vi "AlliGator Phasor Plot Context Menu Handler.vi"(8 "Error In":errorcluster, 11 "Image Event":T1) -> (0 "Error Out":errorcluster, 1 "Message":string, 3 "AlliGator Actions":T4[](array[typedef]))   [LabVIEW 2021, in "AlliGator Phasor Plot.lvlib"]
doc: "Phasor Plot image context menu handler."
uses:
  AlliGator Phasor Plot.lvlib
  Action Engine/AlliGator Q Element.ctl
  Action Engine/AlliGator Q Event.ctl
  Image/Image Display Event.ctl
  Image/Image Control Refnum.ctl
  <vilib>/Utility/miscctls.llb/LVPoint32TypeDef.ctl
  Image/Image Display to Clipboard Options.ctl
  Settings/AlliGator Phasor Plot Graphics Options.ctl
  Settings/AlliGator Settings List.ctl
  ROIs/AlliGator ROI Manager Actions.ctl
  ROIs/AlliGator Selected ROI.ctl
  Image/Image Control ROI Description.ctl
  GUI/AlliGator Windows List.ctl
  AlliGator Phasor Harmonic Manager Actions.ctl
  Phasor Plot Color Map/AlliGator Phasor Color Map Picker.vi
  Variant/Variant to Data/Variant to Boolean.vi
  ROIs/AlliGator Phasor Plot ROI Manager.vi
  Action Engine/AlliGator Action Engine.lvlib
  Image/Image.lvlib
  Settings/AlliGator Settings.lvlib
  Variant/Variant to Data/Variant to Data.lvlib
  Utilities/Utilities.lvlib
  Phasor Plot Color Map/AlliGator Phasor Plot Color Map.lvlib
  ROIs/AlliGator ROIs.lvlib
  GUI/AlliGator GUI.lvlib
  AlliGator Phasor Harmonics.lvlib
  Notebook/Notebook.lvlib
panel:
  # "see the AlliGator License on the block diagram (Ctrl+E or Window:Show Block Diagram)"
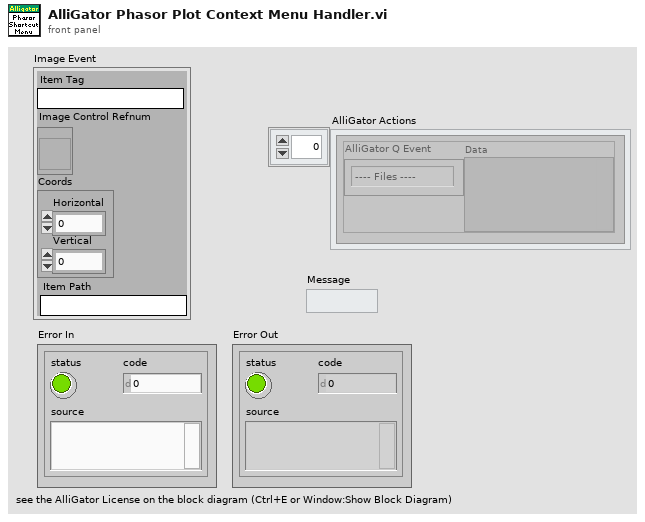
[diagram p1: front panel]
types:
  T1 = typedef "Image.lvlib/Image Display Event.ctl" = cluster{"Item Tag":string, "Image Control Refnum":T2, "Coords":T3, "Item Path":string}
  T2 = typedef "Image.lvlib/Image Control Refnum.ctl" = refnum<vi>
  T3 = typedef "LVPoint32TypeDef.ctl" = cluster{"Horizontal":i32, "Vertical":i32}
  T4 = typedef "AlliGator Action Engine.lvlib/AlliGator Q Element.ctl" = cluster{"AlliGator Q Event":T5, "Data":variant}
  T5 = typedef "AlliGator Action Engine.lvlib/AlliGator Q Event.ctl" = enum16{"---- Files ----", "Files:Set Batch Export Files To Save", "Files:Set Dataset Loading & Pre-processing Options", "Files:Check #Frames in Dataset", "Files:Increment Frame Index", "Files:Open Mask Image", "Files:Open White Light Image", "Files:Open Single Dataset", "Files:New Folder of Folders Selected", "Files:Load File (all Types)_Scriptable", "Files:Move Flattened Series to Folders Series", "Files:Select Folder", "Files:Load FLI Dataset", "Files:Load Swiss SPAD 1 Dataset", "Files:Load Swiss SPAD 2 Dataset", "Files:Load .sdt FLI Dataset", "Files:Load .ptu FLI Dataset", "Files:Load .bin FLI Dataset", "Files:Load Single Gate Image Folder", "Files:Load I/m/phi Dataset (deprecated)", "Files:Load Single Image", "Files:Subtract Background File", "Files:Export FLI Dataset", "Files:Load HDF5 FLI Dataset", "Files:Set Destination File Path", "Files:Save Mask Image", "Files:Batch Conversion", "Files:New Folder Selected", "Files:Close FLI Dataset", "Files:Close FLI Dataset Series", "Files:Close White Light Image", "Files:Close Mask Image", "---- FLI Dataset ----", "FLI Dataset:Channel Arithmetic", "FLI Dataset:Export Average Lifetime Map as ASCII", "FLI Dataset:Export User-Defined Quantity Map as ASCII", "FLI Dataset:Python Function FLI Dataset Event", "FLI Dataset:ROI Analysis", "FLI Dataset:Tilted Logistic Square Gated IRF Characteristics Map", "FLI Dataset:Logistic Square Gated IRF Characteristics Map", "FLI Dataset:Square Gated IRF Characteristics Map", "FLI Dataset:Multi-ROI Single-Pixel Phasor Analysis", "FLI Dataset:Multi-ROI Single-Pixel NLSF Analysis", "FLI Dataset:All ROIs IRF Extraction", "FLI Dataset:All ROIs Decay Fit Non-Interactive (Fast + Individual IRF)", "FLI Dataset:All ROIs Phasor Analysis", "FLI Dataset:All ROIs Decay Fit", "FLI Dataset:Fluorescence Decay Statistics", "FLI Dataset:Update Decay Statistics Graph", "FLI Dataset:Get Decay from ROI", "FLI Dataset:All ROIs Average Lifetimes", "---- FLI Dataset Series ----", "FLI Dataset Series:Sum All Datasets in Series", "FLI Dataset Series:Add Dataset to Accumulated Dataset", "FLI Dataset Series:Display Accumulated Dataset", "FLI Dataset Series:Clear Dataset Series Sum", "FLI Dataset Series:Time-Series Analysis (NLSF)", "FLI Dataset Series:Time-Series Analysis (Phasor)", "---- Image ----", "Image:Update Image Profile Plots", "Image:Image Histogram Cursor Move", "Image:Image Histogram", "Image:Image Contrast", "Image:Set Image Histogram Cursor Move Flag", "Image:Clear Image Overlay", "Image:Use ROI as Search Area", "Image:Set ROI Diameter", "Image:Save Image Data as TIFF", "Image:Save Displayed Image with Overlay", "Image:Save Image Overlay Only", "Image:Save Image as Hot Pixel Mask", "Image:Change Source Image Color Palette", "Image:Copy Image to Clipboard", "Image:Source Image ROI Selection", "Image:Delete All ROIs", "Image:Delete All Unselected ROIs", "Image:Delete ROI", "Image:Merge All ROIs", "Image:Store ROI", "Image:Source Image ROI Storage", "Image:Export ROI Description to Notebook", "Image:Save ROI", "Image:Load ROI", "Image:Paste ROI Definition", "Image:Clear ROI", "Image:Identify ROIs in Mask Image", "Image:Create Complementary ROI", "Image:Create Contour ROI", "Image:Create ROI(s) from Pixels with Peak above Min_Scriptable", "Image:Create ROI(s) from Pixels with Intensity above Min_Scriptable", "Image:Compute ROI Statistics", "Image:Delete ROI(s) based on ROI Characteristics", "Image:Create ROI Grid", "Image:ROI to Individual Pixel ROIs", "Image:Python Function Source Image Event", "Image:Show Phasor Calibration Map ROI Centers", "Image:Convert ROI to Mask Image", "Image:Mouse Move", "Image:Mouse Up", "Image:Set Source Image Mouse Move Flag", "Image:Add Scale Bar Overlay", "Image:Delete Existing ROIs Option", "Image:Overlay ROI Median", "Image:Check Current ROI", "---- Decay ----", "Decay:Clear IRF/Reference Plot", "Decay:Clear Local IRFs", "Decay:Add Decay to Graph", "Decay:Smoothen Plot", "Decay:Smoothen Plot Tail", "Decay:Average Selected Plots", "Decay:Extract IRF", "Decay:Optimal IRF Extraction", "Decay:Threshold IRF", "Decay:Fit to Model IRF", "Decay:Fit IRF to Square Gate", "Decay:Fit IRF to Logistic Square Gate", "Decay:Fit IRF to Tilted Logistic Square Gate", "Decay:Create Bounding Cursors Set", "Decay:Export Bounding Cursors Definition to Notebook", "Decay:Denoise Plot", "Decay:Compute Cumulative Function", "Decay:Use as Reference Decay", "Decay:Show Reference Decay/IRF", "Decay:Extrapolate Decay", "Decay:Create Head & Tail Bounding Cursors", "Decay:Store Cursor-defined Head & Tail Fractions", "Decay:Rebin Plot", "Decay:1-Normalize Decay", "Decay:[0-1]-Normalize Plot", "Decay:Straighten Decay", "Decay:Shift Decay", "Decay:Fold Decay", "Decay:Fit Decay", "Decay:Global Fit of Selected Decays", "Decay:Post Global Fit Script", "Decay:Add Global Fit Parameters to Graph", "Decay:Add Decay Parameter(s) to Plot (Graph)", "Decay:Export Decay to Phasor Graph", "Decay:Plot Decay Shifts", "Decay:Compute Average Lifetime", "Decay:Plot Convolution", "Decay:Graph Tip Strip Update", "---- Decay Statistics ----", "Decay Statistics:Tip Strip Update", "---- Intensity Time Trace ----", "Intensity Time Trace:Use File Timestamp", "Intensity Time Trace:Load Intensity Corrections File", "Intensity Time Trace:Clear Intensity Corrections File", "Intensity Time Trace:Tip Strip Update", "---- Phasor Plot ----", "Phasor Plot:Build Phasor Plot", "Phasor Plot:Change Phasor Plot Color Palette", "Phasor Plot:Adjust Phasor Plot Display Range", "Phasor Plot:Highlight Image ROI in Phasor Plot", "Phasor Plot:Save Phasor Plot Image with Overlay", "Phasor Plot:Export Complex Phasor Map", "Phasor Plot:Export Phasor Ratio Map", "Phasor Plot:Export Average Lifetime Map", "Phasor Plot:Compute Phase Lifetime Histogram", "Phasor Plot:Compute Phasor Ratio Histogram", "Phasor Plot:Compute Phase Lifetime vs Intensity Scatter Plot", "Phasor Plot:Weber 2-Component Decomposition", "Phasor Plot:Update Phasor Color Map Vertices", "Phasor Plot:Clear Phasor Overlay", "Phasor Plot:Use Segment Extremities as References", "Phasor Plot:Use UC/Segment Intersections as References", "Phasor Plot:Use UC/Principal Axis Intersections as References", "Phasor Plot:Use UC/Linear Fit Intersections as References", "Phasor Plot:Update Phasor Plot Reference", "Phasor Plot:Show Local Phasor Info in Phasor Plot", "Phasor Plot:Update Phasor Plot State", "Phasor Plot:Phasor Plot ROI Storage", "Phasor Plot:Phasor Plot ROI Selection", "Phasor Plot:Python Function Phasor Plot Event", "Phasor Plot:Overlay Phasor ROI, Ratio or Map in Source Image", "Phasor Plot:Compute Decay of Selected Phasors", "Phasor Plot:Phasor at Image Pixel", "Phasor Plot:Mouse Move", "Phasor Plot:Mouse Up", "Phasor Plot:Display Range Mouse Move", "Phasor Plot:Set Mouse Move Flag", "---- Phasor Graph ----", "Phasor Graph:Calibrated Phasor Map Series", "Phasor Graph:Whole Image Phasor Scatter Plot (deprecated)", "Phasor Graph:Get Phasor Value", "Phasor Graph:Create New Phasor Plot Dialog", "Phasor Graph:Update Last Phasor Value", "Phasor Graph:Update Phasor (m, phi)", "Phasor Graph:Remove Single Phasor from Plot", "Phasor Graph:Add Single Phasor to Plot", "Phasor Graph:Remove Phasor Plot", "Phasor Graph:Remove Selected Phasor Plots", "Phasor Graph:Clear Phasor Data", "Phasor Graph:Clear Phasor Graph", "Phasor Graph:Cursor Move", "Phasor Graph:Draw Cursor Connecting Line", "Phasor Graph:Clear Cursor Connecting Line", "Phasor Graph:Find UC Intersection", "Phasor Graph:Use UC/Cursor-Defined Line Intersections", "Phasor Graph:Use Selected Plots Fitted Line/UC Intersections", "Phasor Graph:Use Selected Plots Principal Axis/UC Intersections", "Phasor Graph:Show Single Phasor", "Phasor Graph:Save Single Phasor Plot", "Phasor Graph:Save All Phasor Plots", "Phasor Graph:Load Phasor Plot(s)", "Phasor Graph:Phasor Multiplication", "Phasor Graph:Compute Average Phasor", "Phasor Graph:Compute Multiple Average Phasors (Selected Plots)", "Phasor Graph:Export Single Phasor Plot Phase Lifetimes", "Phasor Graph:Phase Lifetime Trajectory", "Phasor Graph:Phase Lifetime vs Intensity Scatter Plot (deprecated)", "Phasor Graph:Parameter 2 vs Parameter 1 Scatter Plot", "Phasor Graph:Use Cursor n Location", "Phasor Graph:Set Reference n to Current Phase Lifetime Value", "Phasor Graph:Set Reference n to Lifetime Value", "Phasor Graph:Set Cursor n Location", "Phasor Graph:Save Phasor Graph Image", "Phasor Graph:Update SEPL Plot", "Phasor Graph:Export Single Phasor Plot Data", "Phasor Graph:Export Selected Phasor Plots Data", "Phasor Graph:Python Function Phasor Graph Event", "Phasor Graph:Tip Strip Update", "---- Calibration ----", "Calibration:Set Calibration Type", "Calibration:Load/Save Phasor Calibration", "Calibration:Load/Save Phasor Calibration Series", "Calibration:Load/Save Phasor Calibration Map", "Calibration:Use as Calibration", "Calibration:Compute Optimal Calibration from Phasor References", "Calibration:Clear Phasor Calibration", "Calibration:Single Phasor Calibration Information", "Calibration:Use as Calibration Series", "Calibration:Use as Calibration Map", "Calibration:Clear Calibration Series", "Calibration:Phasor Calibration Series Information", "Calibration:Clear Calibration Map", "Calibration:Phasor Calibration Map Information", "Calibration:Apply Phasor Calibration", "Calibration:Update Single Plot Calibration", "Calibration:Update Multiple Plots Calibration", "Calibration:Clear Single Plot Calibration", "Calibration:Clear All Plots Calibrations", "Calibration:Clear Plot(s) Calibration(s)?", "Calibration:Phasor Calibration Maps (# Gates Series)", "---- Phasor Ratio ----", "Phasor Ratio:Clear Reference n", "Phasor Ratio:Toggle Selected Plot(s)  Lock to Reference 1", "Phasor Ratio:Use as Reference n", "Phasor Ratio:Send Reference n to Notebook", "Phasor Ratio:Toggle Selected Plot(s)  Lock to Reference 2", "Phasor Ratio:Compute Phasor Ratio at Mouse Location", "Phasor Ratio:Compute Phasor Plot's Average Phasor Ratio", "Phasor Ratio:Compute Time-Series Phasor Ratios", "Phasor Ratio:Fit Line to Phasor Ratio Plot", "Phasor Ratio:Save References", "Phasor Ratio:Load References", "Phasor Ratio:Update Phasor Reference 1", "Phasor Ratio:Update Phasor Reference 2", "Phasor Ratio:Move Cursor n to Reference n", "Phasor Ratio:Use as Phasor Reference 1 Lifetime", "Phasor Ratio:Use as Phasor Reference 2 Lifetime", "Phasor Ratio:Export Phasor Ratio Map as ASCII", "Phasor Ratio:Tip Strip Update", "---- Lifetime & Other Parameters Graph ----", "Lifetime:Tip Strip Update", "---- Decay Fit Parameter Map ----", "Decay Fit Parameter Map:Export ROI NLSF Data as ASCII", "Decay Fit Parameter Map:Set Decay Fit Parameter Map Selection", "Decay Fit Parameter Map:Build Decay Fit Parameter Map", "Decay Fit Parameter Map:Change Decay Fit Parameter Map Color Palette", "Decay Fit Parameter Map:Export Decay Fit Parameter Map Data as ASCII", "Decay Fit Parameter Map:Export All Decay Fit Parameter Maps Data as ASCII", "Decay Fit Parameter Map:Selected Parameter Scatterplot", "Decay Fit Parameter Map:Parameter 2 vs Parameter 1 Scatterplot", "Decay Fit Parameter Map:Save Decay Fit Parameter Map Image", "Decay Fit Parameter Map:Save-Load IRFs & Fit Data", "Decay Fit Parameter Map:Update Local Decay Plots", "Decay Fit Parameter Map:Python Function Decay Fit Parameters Map Event", "Decay Fit Parameter Map:Overlay Decay Fit Parameter Map in Source Image", "Decay Fit Parameter Map:Selected Parameter vs Intensity Scatterplot", "Decay Fit Parameter Map:Mouse Up", "Decay Fit Parameter Map:Display Range Mouse Move", "---- Parameter Map ----", "Parameter Map:Export ROI Parameters Data as ASCII", "Parameter Map:Delete Parameter Map Set", "Parameter Map:Update Parameter List", "Parameter Map:Build Parameter Map", "Parameter Map:Change Parameter Map Color Palette", "Parameter Map:Export Parameter Map Data as ASCII", "Parameter Map:Export All Parameter Maps Data as ASCII", "Parameter Map:Selected Parameter Scatterplot", "Parameter Map:Parameter 2 vs Parameter 1 Scatterplot", "Parameter Map:Selected Parameter vs Intensity Scatterplot", "Parameter Map:Save Parameter Map Image", "Parameter Map:Save-Load IRFs & Parameter Maps (TODO)", "Parameter Map:Set Parameter Map Selection", "Parameter Map:Python Function Parameter Map Event", "Parameter Map:Overlay Parameter Map in Source Image", "Parameter Map:Update Local Decay Plots", "Parameter Map:Mouse Up", "Parameter Map:Display Range Mouse Move", "---- Generic Graph ----", "Generic Graph:Generic XY Graph Event", "Generic Graph:Python Function XY Graph Event", "Generic Graph:New Plot", "Generic Graph:Save Plot", "Generic Graph:XY Plot Histogram", "Generic Graph:Set XY Graph Plot Name", "Generic Graph:Set Last Cursor Style", "Generic Graph:Tip Strip Update", "---- GUI ----", "GUI:Start Script", "GUI:Type of Displayed Image Changed", "GUI:Gate Image Slide Changed", "GUI:Show Busy Icon", "GUI:Show Busy Icon & Abort Button", "GUI:Hide Busy Icon", "GUI:Hide Busy Icon & Abort Button", "GUI:Abort", "GUI:End Script", "GUI:Start Timing", "GUI:End Timing", "GUI:Set State Indicator", "GUI:Send Parameters JSON Strings to Clipboard", "GUI:Set Gate Step", "GUI:Idle", "GUI:Initialization", "GUI:Quit", "GUI:Increment Dataset Index", "GUI:Set Dataset Index to -1", "GUI:Time Series Slider Moved", "GUI:Time Series Slider Changed", "GUI:Toggle Playback or Loop", "GUI:Playback Script", "GUI:Set Phasor Frequency", "GUI:Open Window", "GUI:Start Test Script", "GUI:End Test Script", "DEBUG"}
  T6 = typedef "Image.lvlib/Image Display to Clipboard Options.ctl" = cluster{"Include Overlay (T)":bool, "Image Only (T)":bool}
  T7 = typedef "AlliGator Settings.lvlib/AlliGator Phasor Plot Graphics Options.ctl" = cluster{"UC Color":u32, "Show UC Tau Ticks":bool, "SEPL Color":u32, "Show SEPL Tau Ticks":bool, "Axes Color":u32, "Show (g,s) Ticks":bool, "Show UC":bool, "Show SEPL":bool, "Show Axes":bool, "Show UC Tau Labels":bool, "Show SEPL Tau Labels":bool, "Show (g,s) Labels":bool, "UC Label Size":i16, "UC Label Distance":dbl, "SEPL Label Size":i16, "SEPL Label Distance":dbl, "Axes Label Size":i16, "Axes Label Distance":dbl}
  T8 = typedef "AlliGator ROIs.lvlib/AlliGator ROI Manager Actions.ctl" = enum16{"Undefined", "Delete Current ROI", "Delete All Unselected ROIs", "Delete Multiple ROIs", "Delete All ROIs", "Swap ROIs", "Insert ROI", "Update Current ROI Descriptor", "Rename Current ROI", "Store New ROI", "Store Multiple ROIs", "Select Next ROI", "Select Previous ROI", "Find Selected ROI", "Show All ROIs", "Update ROI Manager Window", "Merge All ROIs", "Unmerge ROI", "Set Selected ROI by ID"}
  T9 = typedef "AlliGator ROIs.lvlib/AlliGator Selected ROI.ctl" = cluster{"Image Ctrl Ref":T2, "All ROIs?":bool}
  T10 = typedef "Image.lvlib/Image Control ROI Description.ctl" = cluster{"Image Control Label":string, "ROI Descriptor":T11}
  T11 = typedef "ROI Descriptor" = cluster{"Global Rectangle":i32[], "Contours":cluster{"ID":enum32{"External", "Internal"}, "Type":u32, "Coordinates":i32[]}[]}
  T12 = typedef "AlliGator GUI.lvlib/AlliGator Windows List.ctl" = enum16{"AlliGator Window", "Settings Window", "Notebook Window", "Dataset Information Window", "Source Image ROI Manager Window", "Phasor Plot ROI Manager Window", "Phasor Harmonic Manager Window", "Histogram Window", "Image Profile Window", "Local Decay Window", "About Window", "Batch Conversion Window", "Shot Noise Influence on Average Lifetime", "Fit Method Benchmark", "AlliGator Alias Definition"}
  T13 = typedef "AlliGator Phasor Plot.lvlib/AlliGator Phasor Harmonic Manager Actions.ctl" = enum16{"Undefined", "Delete Current Harmonic", "Delete Multiple Harmonics", "Delete All Harmonics", "Swap Harmonics", "Insert Harmonics", "Rename Current Harmonic", "Store New Harmonic", "Store Multiple Harmonics", "Select Next Harmonic", "Select Previous Harmonic", "Update Phasor Harmonic Manager Window"}
  T14 = cluster{"Image Control Refnum":T2, "Image to Clipboard Options":T6}
  T15 = typedef "AlliGator Settings.lvlib/AlliGator Settings List.ctl" = enum16{"GUI:Visible Settings Tab", "GUI:Last Run Version", "Source Image:Use Image Histogram for Contrast", "Source Image:Low Count Pixels Rejection Options", "Source Image:High Count Pixels Rejection Options", "Source Image:Use Image Brightness", "Source Image:Blend Overlay with Image Background", "Source Image:Use Fixed ROI Diameter", "Source Image:ROI Diameter", "Source Image:ROI Center Color", "Source Image:Peak Threshold", "Source Image:Intensity Threshold", "Source Image:Image Binning Options", "Source Image:Image Smoothing Options", "Source Image:Image Histogram Active", "Source Image:Invert Binary Mask", "Source Image:Hot Pixel Removal", "Source Image:Overlay Analyzed ROI Center", "Source Image:Auto-Adjust Contrast", "Source Image:Histogram Lower Percentile", "Source Image:Histogram Upper Percentile", "Source Image:Save Source Image", "Source Image:Scale Bar Options", "Source Image:Image Resolution (Pixel Size)", "Source Image:Flatfield Correction", "Source Image:Show Dead Left Columns Correction", "Source Image:Dead Left Columns Correction", "Source Image:Image Pre-Processing Operations Order", "Source Image:Overlay ROI Median", "Source Image:Median Overlay Color", "Data Information:Gate Width", "Data Information:Nanotime Gate Separation", "Data Information:Macrotime Gate Separation", "Data Information:Gate Step", "Data Information:# Gates", "Data Information:Gate Image Exposure", "Data Information:Gate Image Integration", "Data Information:Gates to Skip", "Data Information:Gates to Keep", "Data Information:Define Gates to", "Data Information:Channel Name", "Data Information:Available Channel Names", "Data Information:Channel Arithmetic", "Data Information:Background File Subtraction", "Data Information:Background File", "Data Information:Background Scaling Factor", "Data Information:Background Pile-up Correction", "Data Information:Background Pixel Well Capacity", "Data Information:Laser Period", "Data Information:SYNC Period", "Data Information:Pile-up Correction", "Data Information:Pixel Well Capacity", "Data Information:Dataset Scaling Factor", "Fluorescence Decay_Decay Pre-Processing:Reverse Gates", "Fluorescence Decay_Decay Pre-Processing:Verbose Decay Pre-Processing", "Fluorescence Decay_Decay Pre-Processing:Use Decay Pre-Processing", "Fluorescence Decay_Decay Pre-Processing:Background Subtraction", "Fluorescence Decay_Decay Pre-Processing:Background Definition Range", "Fluorescence Decay_Decay Pre-Processing:Baseline Subtraction Method", "Fluorescence Decay_Decay Pre-Processing:Decay Pre-Processing Operations Order", "Fluorescence Decay_Decay Pre-Processing:Smoothing Parameter", "Fluorescence Decay_Decay Pre-Processing:Shift Decay", "Fluorescence Decay_Decay Pre-Processing:Decay Shift Parameters", "Fluorescence Decay_Decay Pre-Processing:Fold Decay", "Fluorescence Decay_Decay Pre-Processing:# Folds", "Fluorescence Decay_Decay Pre-Processing:1-Normalize Decay", "Fluorescence Decay_Decay Pre-Processing:[0-1]-Normalize Decay", "Fluorescence Decay_Decay Pre-Processing:Smoothen Decay", "Fluorescence Decay_Decay Pre-Processing:Extrapolate Decay", "Fluorescence Decay_Decay Pre-Processing:Use Periodicity", "Fluorescence Decay_Decay Pre-Processing:Use Cursors", "Fluorescence Decay_Decay Pre-Processing:Tail Fraction", "Fluorescence Decay_Decay Pre-Processing:Head Fraction", "Fluorescence Decay_Decay Pre-Processing:Additional Points", "Fluorescence Decay_Decay Pre-Processing:Straighten Decay", "Fluorescence Decay_Decay Pre-Processing:Constant Background", "Fluorescence Decay_Decay Pre-Processing:Pixel-Normalize Decay", "Fluorescence Decay_Advanced Analysis:Extract IRF instead of Decay", "Fluorescence Decay_Advanced Analysis:IRF Extraction Options", "Fluorescence Decay_Advanced Analysis:IRF Optimization Options", "Fluorescence Decay_Advanced Analysis:Square Pulse Options", "Fluorescence Decay_Advanced Analysis:IRF Order", "Fluorescence Decay_Advanced Analysis:IRF Time Constants", "Fluorescence Decay_Advanced Analysis:Wavelet Analysis Options", "Fluorescence Decay_Advanced Analysis:Average Lifetime Options", "Fluorescence Decay_Fit Options:Fit Options", "Fluorescence Decay_Fit Options:Use Legacy Fitting Approach", "Fluorescence Decay_Fit Options:Use Data Information Laser Period", "Fluorescence Decay_Fit Parameters:Displayed Fit Parameters", "Fluorescence Decay_Fit Parameters:Fit Parameter Constraints", "Fluorescence Decay_Fit Parameters:Export Tabulated Results", "Fluorescence Decay_Fit Parameters:MLE Baseline Offset Type", "Fluorescence Decay_Fit Parameters:MLE Baseline Offset", "Fluorescence Decay_Fit Parameters:Guess Parameter Names", "Fluorescence Decay_Fit Parameters:Guess Parameter Values", "Fluorescence Decay_Fit Parameters:Guess Parameters Options", "Fluorescence Decay_Styles:Show Last Decay Only", "Fluorescence Decay_Styles:Decay Graph Color Array", "Fluorescence Decay:Decay Graph Active", "Fluorescence Decay Statistics:Min Peak Value", "Fluorescence Decay Statistics:Reject Low Decay Peak Pixels", "Fluorescence Decay Statistics:Reject High Decay Peak Pixels", "Fluorescence Decay Statistics:Max Peak Value", "Time Traces:Use File Timestamp", "Time Traces:Time Step", "Time Traces:Use Intensity Correction File", "Time Traces:Intensity Correction File", "Phasor Plot:Phasor Plot Smoothing Options", "Phasor Plot:Phasor Plot Size", "Phasor Plot:Phasor Plot Graphics Options", "Phasor Plot:Cumulative Phasor Plot", "Phasor Plot:Use Phasor Brightness", "Phasor Plot:Blend Overlay with Phasor Background", "Phasor Plot:Save Phasor Plot", "Phasor Plot:Show References", "Phasor Plot:Phasor Ratio Decay Range", "Phasor Plot:Exponential Fading", "Phasor Plot:Phasor Ratio Reference Colors", "Phasor Plot:Reference Radius", "Phasor Plot:Show Color Map Vertices", "Phasor Plot:Phasor Plot Active", "Phasor Plot:Phasor Ratio Color Map Type", "Phasor Plot:Phasor Ratio Color Map", "Phasor Plot:Phasor Ratio Display Range", "Phasor Plot:Selected Image ROI(s)", "Phasor Plot:All Image ROIs", "Phasor Plot:Selected Phasor Plot ROI(s)", "Phasor Plot:All Phasor Plot ROIs", "Phasor Plot:Phasor Ratio Color-Coded Quantity", "Phasor Plot:Store Phasor Harmonics", "Phasor Plot:Draw Reference Segment", "Phasor Plot:User-Defined Quantity", "Phasor Graph:Phasor Frequency", "Phasor Graph:Phasor Ratio Type", "Phasor Graph:Pixel-level Phasor Computation", "Phasor Graph:Save Phasor Graph", "Phasor Graph:Phasor Graph Active", "Phasor Graph:Phasor SDV Options", "Phasor Calibration:Use Backup Calibration if needed", "Phasor Graph:Define Shortest Lifetime as", "Phasor Calibration:Backup Calibration Type", "Phasor Calibration:Calibration Type", "Phasor Calibration:Calibration Lifetime", "Phasor Calibration:Calibration Map Algorithm", "Single-Exponential Phasor Locus (SEPL):Gate Parameters", "Single-Exponential Phasor Locus (SEPL):User-defined Gate", "Single-Exponential Phasor Locus (SEPL):User-defined IRF", "Single-Exponential Phasor Locus (SEPL):Phasor Parameters", "Single-Exponential Phasor Locus (SEPL):Decay & IRF Parameters", "Single-Exponential Phasor Locus (SEPL):Display Parameters", "Lifetime Analysis:Decay Analysis Parameters", "Lifetime Analysis:Lifetime Map Active", "Plugins:Python Settings", "Miscellaneous:Verbose Mode", "Miscellaneous:Beep after Script", "Miscellaneous:Saved Image File Format", "Miscellaneous:Exported Gate Image Settings", "Miscellaneous:Include Loading in Timing", "Miscellaneous:Verbose Settings Mode", "Miscellaneous:Histogram Options", "Miscellaneous:Beep on Error", "Miscellaneous:# Logical Processors Used", "Miscellaneous:ROI Description Max Characters", "Miscellaneous:Verbose Error Mode", "Miscellaneous:Transparent Mask Color"}
  T16 = cluster{"Global Rectangle":i32[], "Contours":cluster{"Contour Type":u32, "ROI Type":u32, "Points":i32[]}[]}
  T17 = typedef "Image.lvlib/Image Point.ctl" = cluster{"X":i32, "Y":i32}
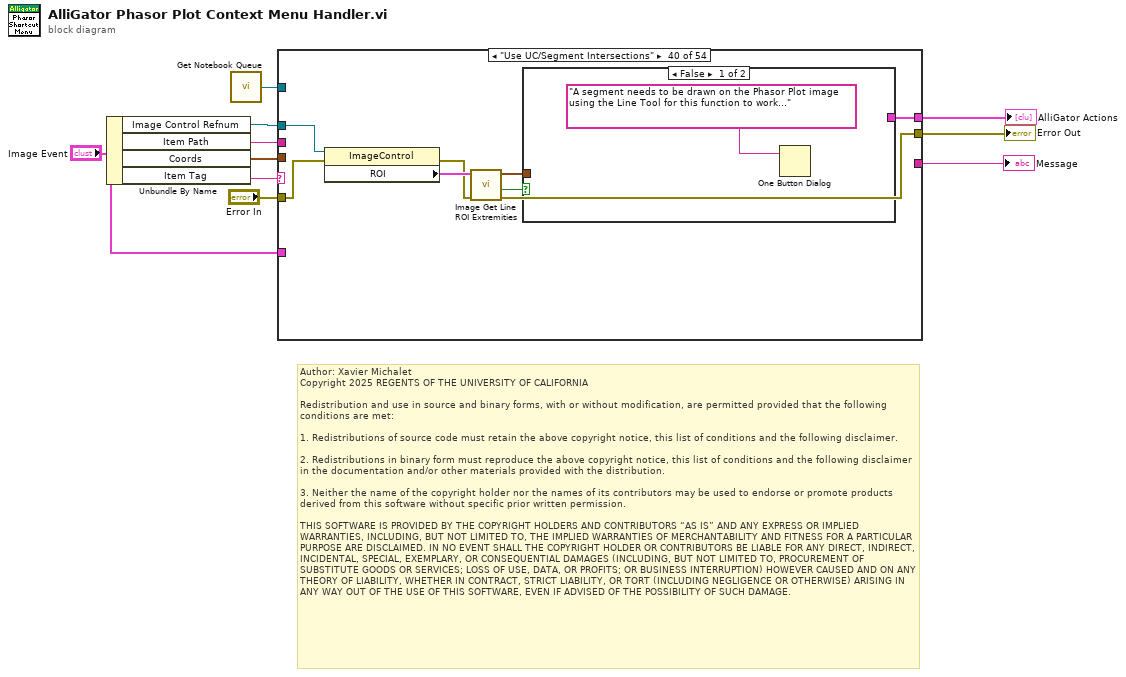
[diagram p0: block diagram]
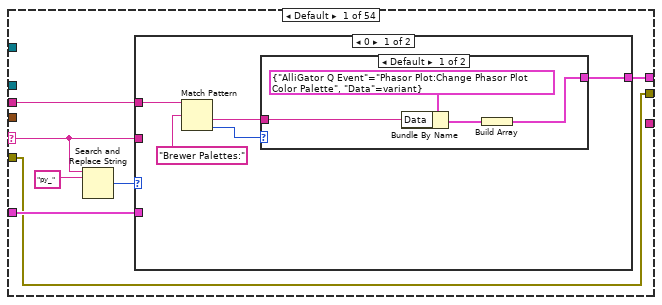
[diagram p2: hidden frame]
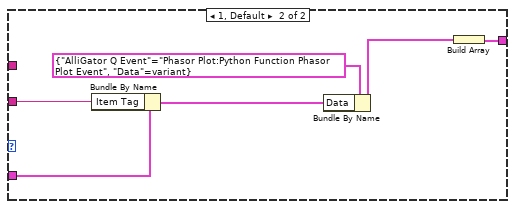
[diagram p4: hidden frame]
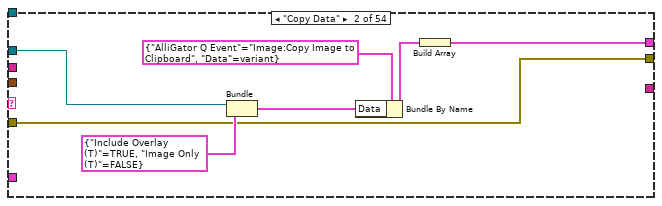
[diagram p5: hidden frame]
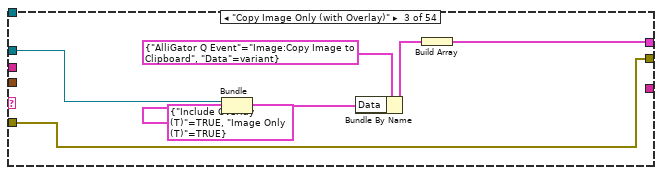
[diagram p6: hidden frame]
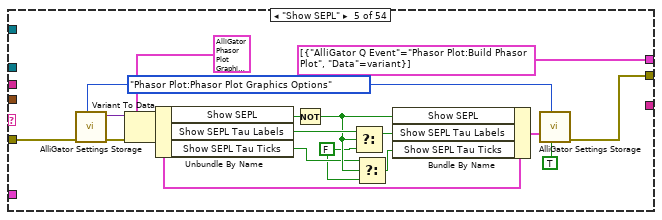
[diagram p8: hidden frame]
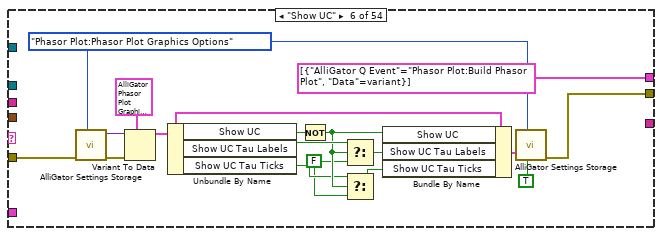
[diagram p9: hidden frame]
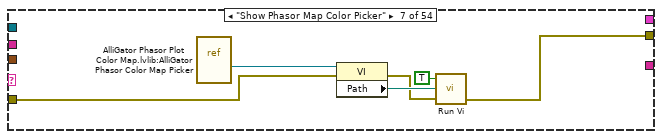
[diagram p10: hidden frame]
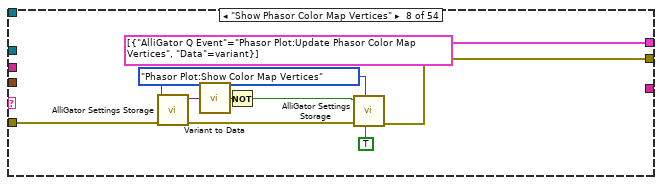
[diagram p11: hidden frame]
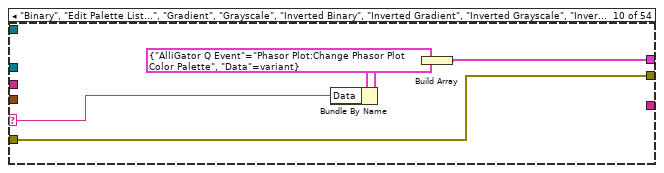
[diagram p13: hidden frame]
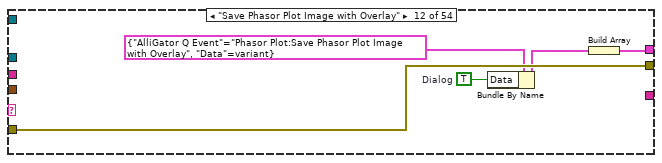
[diagram p15: hidden frame]
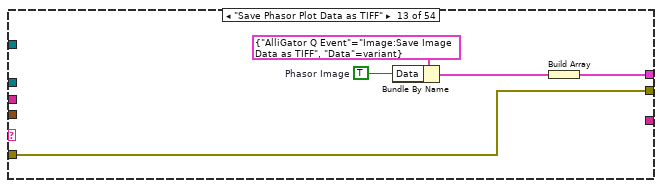
[diagram p16: hidden frame]
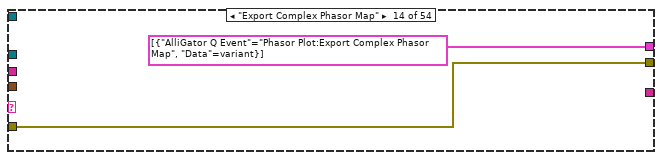
[diagram p17: hidden frame]
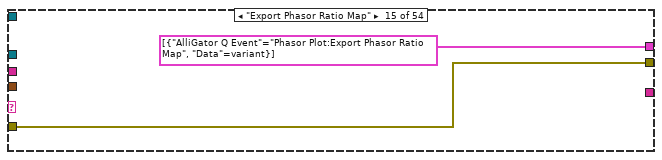
[diagram p18: hidden frame]
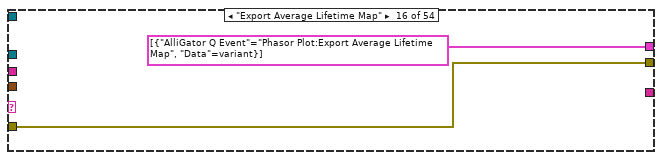
[diagram p19: hidden frame]
diagram:
  # "Author: Xavier Michalet\nCopyright 2025 REGENTS OF THE UNIVERSITY OF CALIFORNIA\n\nRedistribution and use in source and binary forms, with or without modification, are permitted provided that the following conditions are met:\n\n1. Redistributions of source code must retain the above copyright notice, this list of conditions and the following disclaimer.\n\n2. Redistributions in binary form must reproduce the above copyright notice, this list of conditions and the following disclaimer in the documentation and/or other materials provided with the distribution.\n\n3. Neither the name of the copyright holder nor the names of its contributors may be used to endorse or promote products derived from this software without specific prior written permission.\n\nTHIS SOFTWARE IS PROVIDED BY THE COPYRIGHT HOLDERS AND CONTRIBUTORS “AS IS” AND ANY EXPRESS OR IMPLIED WARRANTIES, INCLUDING, BUT NOT LIMITED TO, THE IMPLIED WARRANTIES OF MERCHANTABILITY AND FITNESS FOR A PARTICULAR PURPOSE ARE DISCLAIMED. IN NO EVENT SHALL THE COPYRIGHT HOLDER OR CONTRIBUTORS BE LIABLE FOR ANY DIRECT, INDIRECT, INCIDENTAL, SPECIAL, EXEMPLARY, OR CONSEQUENTIAL DAMAGES (INCLUDING, BUT NOT LIMITED TO, PROCUREMENT OF SUBSTITUTE GOODS OR SERVICES; LOSS OF USE, DATA, OR PROFITS; OR BUSINESS INTERRUPTION) HOWEVER CAUSED AND ON ANY THEORY OF LIABILITY, WHETHER IN CONTRACT, STRICT LIABILITY, OR TORT (INCLUDING NEGLIGENCE OR OTHERWISE) ARISING IN ANY WAY OUT OF THE USE OF THIS SOFTWARE, EVEN IF ADVISED OF THE POSSIBILITY OF SUCH DAMAGE."
  n1 = Unbundle By Name("Image Event") -> ("Image Control Refnum"=w3:T2, "Item Path"=w6:string, "Coords"=w5:T3, "Item Tag"=w4:string)
  n2 = call "Get Notebook Queue.vi"() -> ("Notebook Queue"=w8:refnum<queue>)  [unwired: 9 in]
  n3 = case shown="\"Use UC/Segment Intersections\"" w4 {
    selector: w4 -> [w11 _ _ _ _ _ _ _ _ w100 _ _ _ _ _ _ _ _ w129 _ w144 _ _ _ _ _ _ _ _ _ _ _ _ _ _ _ _ _ _ _ _ _ _ _ _ _ _ _ _ _ _ _ _ _]
    tunnel: w3 -> [_ w35 w42 _ _ _ _ _ _ _ _ _ _ _ _ _ _ _ _ w140 _ w160 w168 w173 _ w181 _ _ _ _ _ _ _ _ _ _ _ _ w229 w241 _ _ _ _ _ _ _ _ _ _ _ _ w311 w314]
    tunnel: w6 -> [w17 _ _ _ _ _ _ _ _ _ _ _ _ _ _ _ _ _ _ _ _ _ _ _ _ _ _ _ _ _ _ _ _ _ _ _ _ _ _ _ _ _ _ _ _ _ _ _ _ _ _ _ _ _]
    tunnel: w5 -> [_ _ _ _ _ _ _ _ _ _ _ _ _ _ _ _ _ _ _ _ _ _ _ _ _ _ _ _ _ _ _ _ _ _ _ _ _ _ _ _ _ _ _ _ _ _ _ _ _ _ _ _ _ _]
    tunnel: "Error In" -> [w12 w33 w40 w47 w62 w79 w83 w90 w97 w98 w103 w108 w113 w114 w116 w118 w120 w122 w133 w137 w145 w156 w164 w171 w177 w178 w188 w190 w197 w201 w202 w204 w206 w208 w210 w211 w216 w221 w224 w236 w249 w254 w258 w263 w269 w276 w282 w284 w289 w294 w297 w307 w309 w313]
    tunnel: [w16 w34 w41 _ T4[] [{"AlliGator Q Event"=enum."Phasor Plot:Build Phasor Plot", "Data"=variant}] ("element") T4[] [{"AlliGator Q Event"=enum."Phasor Plot:Build Phasor Plot", "Data"=variant}] ("element") _ T4[] [{"AlliGator Q Event"=enum."Phasor Plot:Update Phasor Color Map Vertices", "Data"=variant}] ("element") _ w99 _ w105 w111 T4[] [{"AlliGator Q Event"=enum."Phasor Plot:Export Complex Phasor Map", "Data"=variant}] ("element") T4[] [{"AlliGator Q Event"=enum."Phasor Plot:Export Phasor Ratio Map", "Data"=variant}] ("element") T4[] [{"AlliGator Q Event"=enum."Phasor Plot:Export Average Lifetime Map", "Data"=variant}] ("element") _ _ w130 w138 w146 w157 w165 w172 T4[] [{"AlliGator Q Event"=enum."Image:Paste ROI Definition", "Data"=variant}] ("element") w180 _ _ _ _ _ T4[] [{"AlliGator Q Event"=enum."Phasor Plot:Compute Phase Lifetime Histogram", "Data"=variant}] ("element") T4[] [{"AlliGator Q Event"=enum."Phasor Plot:Compute Phasor Ratio Histogram", "Data"=variant}] ("element") T4[] [{"AlliGator Q Event"=enum."Phasor Plot:Compute Phase Lifetime vs Intensity Scatter Plot", "Data"=variant}] ("element") T4[] [{"AlliGator Q Event"=enum."Phasor Plot:Weber 2-Component Decomposition", "Data"=variant}] ("element") _ w213 w218 w223 w235 w251 w256 w259 w265 w271 w273 T4[] [{"AlliGator Q Event"=enum."Phasor Ratio:Save References", "Data"=variant}] ("element") T4[] [{"AlliGator Q Event"=enum."Phasor Ratio:Load References", "Data"=variant}] ("element") w285 w290 w296 _ _ _] -> w9
    tunnel: [w12 w33 w40 w47 w60 w77 w82 w88 w97 w98 w103 w108 w113 w114 w116 w118 w120 w121 w133 w137 w145 w156 w164 w171 w177 w179 w188 w189 w195 w199 w202 w204 w206 w208 w210 w211 w216 w221 w222 w234 w249 w254 w258 w263 w269 w276 w282 w284 w289 w294 w295 w307 w308 w312] -> w7
    tunnel: w8 -> [_ _ _ _ _ _ _ _ _ _ _ _ _ _ _ _ _ _ _ _ _ _ _ _ _ _ _ _ _ _ _ _ _ _ _ _ _ _ _ _ _ _ _ _ _ _ _ _ _ _ _ _ _ _]
    tunnel: "Image Event" -> [w13 _ _ _ _ _ _ _ _ _ _ _ _ _ _ _ _ _ _ _ _ _ _ _ _ _ _ _ _ _ _ _ _ _ _ _ _ _ _ _ _ _ _ _ _ _ _ _ _ _ _ _ _ _]
    tunnel: [_ _ _ _ _ _ _ _ _ _ _ _ _ _ _ _ _ _ _ _ _ _ _ _ _ _ _ _ w194 w198 _ _ _ _ _ _ _ _ _ _ _ _ _ _ _ _ _ _ _ _ _ _ _ _] -> w1
    frame Default {
      n4 = Search and Replace String(input string=w11, search string="py_") -> (number of replacements=w14:i32)  [unwired: 6 in, 3 out]
      n5 = case shown="0" w14 {
        tunnel: w17 -> [w19 _]
        tunnel: [w18 w27] -> w16
        tunnel: w11 -> [_ w29]
        tunnel: w13 -> [_ w28]
        frame 0 {
          n6 = Match Pattern(string=w19, regular expression="Brewer Palettes:") -> (after substring=w20:string, offset past match=w21:i32)  [unwired: 1 in, 2 out]
          n7 = case shown="Default" w21 {
            tunnel: w20 -> [w24 _]
            tunnel: [w23 _] -> w18
            frame Default {
              n8 = Bundle By Name(cluster=T4 {"AlliGator Q Event"=enum."Phasor Plot:Change Phasor Plot Color Palette", "Data"=variant} ("element"), "Data"=w24) -> (w25:T4)
              n9 = Build Array(w25) -> (w23:T4[])
            }
            frame -1 {
            }
          }
        }
        frame 1, Default {
          n10 = Bundle By Name(cluster=w28, "Item Tag"=w29) -> (w32:T1)
          n11 = Bundle By Name(cluster=T4 {"AlliGator Q Event"=enum."Phasor Plot:Python Function Phasor Plot Event", "Data"=variant}, "Data"=w32) -> (w31:T4)
          n12 = Build Array(w31) -> (w27:T4[])
        }
      }
    }
    frame "Copy Data" {
      n13 = Bundle("Image Control Refnum"=w35, "Image to Clipboard Options"=T6 {"Include Overlay (T)"=TRUE, "Image Only (T)"=FALSE}) -> (w36:T14)  [unwired: 1 in]
      n14 = Bundle By Name(cluster=T4 {"AlliGator Q Event"=enum."Image:Copy Image to Clipboard", "Data"=variant} ("element"), "Data"=w36) -> (w38:T4)
      n15 = Build Array(w38) -> (w34:T4[])
    }
    frame "Copy Image Only (with Overlay)" {
      n16 = Bundle("Image Control Refnum"=w42, "Image to Clipboard Options"=T6 {"Include Overlay (T)"=TRUE, "Image Only (T)"=TRUE}) -> (w43:T14)  [unwired: 1 in]
      n17 = Bundle By Name(cluster=T4 {"AlliGator Q Event"=enum."Image:Copy Image to Clipboard", "Data"=variant} ("element"), "Data"=w43) -> (w45:T4)
      n18 = Build Array(w45) -> (w41:T4[])
    }
    frame "-----------------------" {
    }
    frame "Show SEPL" {
      w49 = FALSE ("f")
      w63 = AlliGator_Settings_List."Phasor Plot:Phasor Plot Graphics Options" ("AlliGator Settings List")
      n19 = call "AlliGator Settings Storage.vi"("AlliGator Settings List"=w63, "Error In"=w62) -> ("Error Out"=w58:errorcluster, "Variant Data out"=w59:variant)  [unwired: 8 in]
      n20 = Variant To Data(error in=w58, type=T7 {"UC Color"=3381759, "Show UC Tau Ticks"=TRUE, "SEPL Color"=3381759, "Show SEPL Tau Ticks"=TRUE, "Axes Color"=16776960, "Show (g,s) Ticks"=FALSE, "Show UC"=FALSE, "Show SEPL"=TRUE, "Show Axes"=FALSE, "Show UC Tau Labels"=FALSE, "Show SEPL Tau Labels"=FALSE, "Show (g,s) Labels"=FALSE, "UC Label Size"=18, "UC Label Distance"=0.0, "SEPL Label Size"=18, "SEPL Label Distance"=0.0, "Axes Label Size"=18, "Axes Label Distance"=0.0} ("Phasor Plot Graphics Options"), Variant=w59) -> (data=w55:T7)  [unwired: 1 out]
      n21 = Unbundle By Name(w55) -> ("Show SEPL"=w56:bool, "Show SEPL Tau Labels"=w53:bool, "Show SEPL Tau Ticks"=w50:bool)
      n22 = Not(x=w56) -> (.not. x?=w51:bool)
      n23 = Select(t=w53, s=w51, f=w49) -> (s? t:f=w52:bool)
      n24 = Select(t=w50, s=w51, f=w49) -> (s? t:f=w48:bool)
      n25 = Bundle By Name(cluster=w55, "Show SEPL"=w51, "Show SEPL Tau Labels"=w52, "Show SEPL Tau Ticks"=w48) -> (w54:T7)
      n26 = call "AlliGator Settings Storage.vi"("Get(F)/Set"=TRUE, "AlliGator Settings List"=w63, "Variant Data in"=w54) -> ("Error Out"=w60:errorcluster)  [unwired: 7 in, 1 out]
    }
    frame "Show UC" {
      w66 = FALSE ("f")
      w80 = AlliGator_Settings_List."Phasor Plot:Phasor Plot Graphics Options" ("AlliGator Settings List")
      n27 = call "AlliGator Settings Storage.vi"("AlliGator Settings List"=w80, "Error In"=w79) -> ("Error Out"=w75:errorcluster, "Variant Data out"=w76:variant)  [unwired: 8 in]
      n28 = Variant To Data(error in=w75, type=T7 {"UC Color"=3381759, "Show UC Tau Ticks"=TRUE, "SEPL Color"=3381759, "Show SEPL Tau Ticks"=TRUE, "Axes Color"=16776960, "Show (g,s) Ticks"=FALSE, "Show UC"=FALSE, "Show SEPL"=TRUE, "Show Axes"=FALSE, "Show UC Tau Labels"=FALSE, "Show SEPL Tau Labels"=FALSE, "Show (g,s) Labels"=FALSE, "UC Label Size"=18, "UC Label Distance"=0.0, "SEPL Label Size"=18, "SEPL Label Distance"=0.0, "Axes Label Size"=18, "Axes Label Distance"=0.0} ("Phasor Plot Graphics Options"), Variant=w76) -> (data=w72:T7)  [unwired: 1 out]
      n29 = Unbundle By Name(w72) -> ("Show UC"=w73:bool, "Show UC Tau Labels"=w70:bool, "Show UC Tau Ticks"=w67:bool)
      n30 = Not(x=w73) -> (.not. x?=w68:bool)
      n31 = Select(t=w70, s=w68, f=w66) -> (s? t:f=w69:bool)
      n32 = Select(t=w67, s=w68, f=w66) -> (s? t:f=w65:bool)
      n33 = Bundle By Name(cluster=w72, "Show UC"=w68, "Show UC Tau Labels"=w69, "Show UC Tau Ticks"=w65) -> (w71:T7)
      n34 = call "AlliGator Settings Storage.vi"("Get(F)/Set"=TRUE, "AlliGator Settings List"=w80, "Variant Data in"=w71) -> ("Error Out"=w77:errorcluster)  [unwired: 7 in, 1 out]
    }
    frame "Show Phasor Map Color Picker" {
      n35 = vi-ref "AlliGator Phasor Plot Color Map.lvlib:AlliGator Phasor Color Map Picker.vi"() -> (w87:refnum<vi>)
      n36 = property class="VI"(reference=w87, error in=w83) -> (error out=w85:errorcluster, "Path"=w86:path)  [unwired: 1 out]
      n37 = call "Run Vi.vi"("Bring To Front (T)"=TRUE, "VI Path"=w86, "error in (no error)"=w85) -> ("error out"=w82:errorcluster)  [unwired: 5 in, 1 out]
    }
    frame "Show Phasor Color Map Vertices" {
      w95 = AlliGator_Settings_List."Phasor Plot:Show Color Map Vertices" ("AlliGator Settings List")
      n38 = call "AlliGator Settings Storage.vi"("AlliGator Settings List"=w95, "Error In"=w90) -> ("Error Out"=w96:errorcluster, "Variant Data out"=w94:variant)  [unwired: 8 in]
      n39 = call-poly "Variant to Data.vi"("Variant"=w94) -> ("Value"=w93:bool)  [unwired: 8 in]
      n40 = Not(x=w93) -> (.not. x?=w92:bool)
      n41 = call "AlliGator Settings Storage.vi"("Get(F)/Set"=TRUE, "AlliGator Settings List"=w95, "Error In"=w96, "Variant Data in"=w92) -> ("Error Out"=w88:errorcluster)  [unwired: 6 in, 1 out]
    }
    frame "---------Palette----------" {
    }
    frame "Binary", "Edit Palette List...", "Gradient", "Grayscale", "Inverted Binary", "Inverted Gradient", "Inverted Grayscale", "Inverted Rainvow", "Inverted Temperature", "Rainbow", "Refresh Image", "Select New Palette...", "Temperature" {
      n42 = Bundle By Name(cluster=T4 {"AlliGator Q Event"=enum."Phasor Plot:Change Phasor Plot Color Palette", "Data"=variant} ("element"), "Data"=w100) -> (w101:T4)
      n43 = Build Array(w101) -> (w99:T4[])
    }
    frame "--------- Others  ---------" {
    }
    frame "Save Phasor Plot Image with Overlay" {
      w104 = TRUE  # Dialog
      n44 = Bundle By Name(cluster=T4 {"AlliGator Q Event"=enum."Phasor Plot:Save Phasor Plot Image with Overlay", "Data"=variant} ("Time-Gated Phasor Q Element"), "Data"=w104) -> (w106:T4)
      n45 = Build Array(w106) -> (w105:T4[])
    }
    frame "Save Phasor Plot Data as TIFF" {
      w109 = TRUE  # Phasor Image
      n46 = Bundle By Name(cluster=T4 {"AlliGator Q Event"=enum."Image:Save Image Data as TIFF", "Data"=variant} ("Time-Gated Phasor Q Element"), "Data"=w109) -> (w112:T4)
      n47 = Build Array(w112) -> (w111:T4[])
    }
    frame "Export Complex Phasor Map" {
    }
    frame "Export Phasor Ratio Map" {
    }
    frame "Export Average Lifetime Map" {
    }
    frame "----------- ROIs ---------------" {
    }
    frame "Phasor Plot ROI Manager" {
      n48 = vi-ref "AlliGator ROIs.lvlib:AlliGator Phasor Plot ROI Manager.vi"() -> (w125:refnum<vi>)
      n49 = property class="VI"(reference=w125, error in=w122) -> (error out=w123:errorcluster, "Path"=w124:path)  [unwired: 1 out]
      n50 = call "Run Vi.vi"("VI Path"=w124, "error in (no error)"=w123) -> ("error out"=w121:errorcluster)  [unwired: 6 in, 1 out]
    }
    frame "Next ROI", "Previous ROI", "Show All ROIs" {
      n51 = case shown="\"Previous ROI\"" w129 {
        tunnel: [AlliGator_ROI_Manager_Actions."Show All ROIs" ("Action") AlliGator_ROI_Manager_Actions."Select Next ROI" ("Action") AlliGator_ROI_Manager_Actions."Select Previous ROI" ("Action")] -> w127
        frame "Show All ROIs", Default {
        }
        frame "Next ROI" {
        }
        frame "Previous ROI" {
        }
      }
      n52 = Bundle("Action"=w127, -1) -> (w126:cluster{"Action":T8, i32})  [unwired: 1 in]
      n53 = Bundle By Name(cluster=T4 {"AlliGator Q Event"=enum."Phasor Plot:Phasor Plot ROI Selection", "Data"=variant} ("element"), "Data"=w126) -> (w131:T4)
      n54 = Build Array(w131) -> (w130:T4[])
    }
    frame "Hide All ROIs" {
      n55 = property class="ImageControl"(reference=w140) -> ("Label.Text"=w139:string)  [unwired: 1 in, 2 out]
      n56 = Bundle By Name(cluster=T4 {"AlliGator Q Event"=enum."Image:Clear ROI", "Data"=variant} ("element"), "Data"=w139) -> (w141:T4)
      n57 = Build Array(w141) -> (w138:T4[])
    }
    frame "Delete All ROIs", "Delete All Unselected ROIs", "Delete ROI", "Merge All ROIs", "Store ROI", "Unmerge ROI" {
      n58 = case shown="\"Delete All Unselected ROIs\"" w144 {
        tunnel: [AlliGator_ROI_Manager_Actions."Store New ROI" ("Action") AlliGator_ROI_Manager_Actions."Delete Current ROI" ("Action") AlliGator_ROI_Manager_Actions."Delete All Unselected ROIs" ("Action") AlliGator_ROI_Manager_Actions."Delete All ROIs" ("Action") AlliGator_ROI_Manager_Actions."Merge All ROIs" ("Action") AlliGator_ROI_Manager_Actions."Unmerge ROI" ("Action")] -> w143
        frame "Store ROI", Default {
        }
        frame "Delete ROI" {
        }
        frame "Delete All Unselected ROIs" {
        }
        frame "Delete All ROIs" {
        }
        frame "Merge All ROIs" {
        }
        frame "Unmerge ROI" {
        }
      }
      n59 = Bundle By Name(cluster=T4 {"AlliGator Q Event"=enum."Phasor Plot:Phasor Plot ROI Storage", "Data"=variant} ("element"), "Data"=w143) -> (w147:T4)
      n60 = Build Array(w147) -> (w146:T4[])
    }
    frame "Save Current ROI" {
      n61 = Bundle(cluster=T9 {"Image Ctrl Ref"=refnum, "All ROIs?"=TRUE} ("Selected ROI"), "Image Ctrl Ref"=w160, "All ROIs?"=FALSE ("create if not found? (F)")) -> (w159:T9)
      n62 = Bundle By Name(cluster=T4 {"AlliGator Q Event"=enum."Image:Save ROI", "Data"=variant} ("element"), "Data"=w159) -> (w161:T4)
      n63 = Build Array(w161) -> (w157:T4[])
    }
    frame "Save All ROIs" {
      n64 = Bundle(cluster=T9 {"Image Ctrl Ref"=refnum, "All ROIs?"=TRUE} ("Selected ROI"), "Image Ctrl Ref"=w168, "All ROIs?"=TRUE ("create if not found? (F)")) -> (w167:T9)
      n65 = Bundle By Name(cluster=T4 {"AlliGator Q Event"=enum."Image:Save ROI", "Data"=variant} ("element"), "Data"=w167) -> (w169:T4)
      n66 = Build Array(w169) -> (w165:T4[])
    }
    frame "Load ROI(s)" {
      n67 = Bundle By Name(cluster=T4 {"AlliGator Q Event"=enum."Image:Load ROI", "Data"=variant} ("element"), "Data"=w173) -> (w174:T4)
      n68 = Build Array(w174) -> (w172:T4[])
    }
    frame "Paste ROI Definitions" {
    }
    frame "Export ROI Description to Notebook" {
      n69 = property class="ImageControl"(reference=w181, error in=w178) -> (error out=w179:errorcluster, "Label.Text"=w185:string, "ROI"=w184:T16)  [unwired: 1 out]
      n70 = Bundle By Name(cluster=T10 {"Image Control Label"="", "ROI Descriptor"={"Global Rectangle"=[], "Contours"=[]}}, "Image Control Label"=w185, "ROI Descriptor"=w184) -> (w182:T10)
      n71 = Bundle By Name(cluster=T4 {"AlliGator Q Event"=enum."Image:Export ROI Description to Notebook", "Data"=variant} ("element"), "Data"=w182) -> (w186:T4)
      n72 = Build Array(w186) -> (w180:T4[])
    }
    frame "----------- Phasor Harmonic Manager -----------" {
    }
    frame "Phasor Harmonic Manager" {
      n73 = call "AlliGator Get Ancillary Window Path.vi"("Error In"=w190, "AlliGator Window"=AlliGator_Windows_List."Phasor Harmonic Manager Window" ("AlliGator Windows")) -> ("Error Out"=w192:errorcluster, "VI Path"=w193:path)  [unwired: 8 in]
      n74 = call "Run Vi.vi"("VI Path"=w193, "error in (no error)"=w192) -> ("error out"=w189:errorcluster)  [unwired: 6 in, 1 out]
    }
    frame "Delete Harmonic" {
      n75 = call "AlliGator Phasor Harmonic Storage [SGL].vi"("Error In"=w197, "Action"=AlliGator_Phasor_Harmonic_Manager_Actions."Delete Current Harmonic") -> ("Error Out"=w195:errorcluster, "Message"=w194:string)  [unwired: 4 in, 4 out]
    }
    frame "Delete All Harmonics" {
      n76 = call "AlliGator Phasor Harmonic Storage [SGL].vi"("Error In"=w201, "Action"=AlliGator_Phasor_Harmonic_Manager_Actions."Delete All Harmonics") -> ("Error Out"=w199:errorcluster, "Message"=w198:string)  [unwired: 4 in, 4 out]
    }
    frame "------------- Analysis ------------" {
    }
    frame "Phase Lifetime Histogram" {
    }
    frame "Phasor Ratio Histogram" {
    }
    frame "Phase Lifetime vs Intensity Scatter Plot" {
    }
    frame "Weber 2-Component Decomposition" {
    }
    frame "----------- Phasor Ratio References -----------" {
    }
    frame "Set Reference 1 to User-entered Lifetime" {
      n77 = Bundle By Name(cluster=T4 {"AlliGator Q Event"=enum."Phasor Graph:Set Reference n to Lifetime Value", "Data"=variant} ("element"), "Data"=1) -> (w214:T4)
      n78 = Build Array(w214) -> (w213:T4[])
    }
    frame "Set Reference 2 to User-entered Lifetime" {
      n79 = Bundle By Name(cluster=T4 {"AlliGator Q Event"=enum."Phasor Graph:Set Reference n to Lifetime Value", "Data"=variant} ("element"), "Data"=2) -> (w219:T4)
      n80 = Build Array(w219) -> (w218:T4[])
    }
    frame "Use Segment Extremities" {
      n81 = property class="ImageControl"(reference=w229, error in=w224) -> (error out=w225:errorcluster, "ROI"=w228:T16)  [unwired: 1 out]
      n82 = call "Image Get Line ROI Extremities.vi"("Error In"=w225, "ROI"=w228) -> ("Error Out"=w222:errorcluster, "Is Line?"=w226:bool, "Line Extremities"=w227:T17[])  [unwired: 7 in]
      n83 = case shown="True" w226 {
        tunnel: w227 -> [_ w231]
        tunnel: [_ w230] -> w223
        frame False {
        }
        frame True {
          n84 = Bundle By Name(cluster=T4 {"AlliGator Q Event"=enum."Phasor Plot:Use Segment Extremities as References", "Data"=variant} ("element"), "Data"=w231) -> (w232:T4)
          n85 = Build Array(w232) -> (w230:T4[])
        }
      }
    }
    frame "Use UC/Segment Intersections" {
      n86 = property class="ImageControl"(reference=w241, error in=w236) -> (error out=w237:errorcluster, "ROI"=w240:T16)  [unwired: 1 out]
      n87 = call "Image Get Line ROI Extremities.vi"("Error In"=w237, "ROI"=w240) -> ("Error Out"=w234:errorcluster, "Is Line?"=w238:bool, "Line Extremities"=w239:T17[])  [unwired: 7 in]
      n88 = case shown="False" w238 {
        tunnel: w239 -> [_ w244]
        tunnel: [_ w243] -> w235
        frame False {
          n89 = One Button Dialog(message="A segment needs to be drawn on the Phasor Plot image using the Line Tool for this function to work...") -> ()  [unwired: 1 in, 1 out]
        }
        frame True {
          n90 = Bundle By Name(cluster=T4 {"AlliGator Q Event"=enum."Phasor Plot:Use UC/Segment Intersections as References", "Data"=variant} ("element"), "Data"=w244) -> (w245:T4)
          n91 = Build Array(w245) -> (w243:T4[])
        }
      }
    }
    frame "Use UC/Major Axis Intersections" {
      n92 = Bundle By Name(cluster=T4 {"AlliGator Q Event"=enum."Phasor Plot:Use UC/Principal Axis Intersections as References", "Data"=variant} ("element"), "Data"=TRUE) -> (w248:T4)
      n93 = Build Array(w248) -> (w251:T4[])
    }
    frame "Use UC/Minor Axis Intersections" {
      n94 = Bundle By Name(cluster=T4 {"AlliGator Q Event"=enum."Phasor Plot:Use UC/Principal Axis Intersections as References", "Data"=variant} ("element"), "Data"=FALSE) -> (w253:T4)
      n95 = Build Array(w253) -> (w256:T4[])
    }
    frame "Use UC/Linear Fit Intersections" {
      n96 = Build Array(T4 {"AlliGator Q Event"=enum."Phasor Plot:Use UC/Linear Fit Intersections as References", "Data"=variant} ("element")) -> (w259:T4[])
    }
    frame "Clear Reference 1" {
      n97 = Bundle By Name(cluster=T4 {"AlliGator Q Event"=enum."Phasor Ratio:Clear Reference n", "Data"=variant} ("element"), "Data"=1) -> (w262:T4)
      n98 = Build Array(w262, T4 {"AlliGator Q Event"=enum."Phasor Plot:Update Phasor Plot Reference", "Data"=variant} ("element")) -> (w265:T4[])
    }
    frame "Clear Reference 2" {
      n99 = Bundle By Name(cluster=T4 {"AlliGator Q Event"=enum."Phasor Ratio:Clear Reference n", "Data"=variant} ("element"), "Data"=2) -> (w268:T4)
      n100 = Build Array(w268, T4 {"AlliGator Q Event"=enum."Phasor Plot:Update Phasor Plot Reference", "Data"=variant} ("element")) -> (w271:T4[])
    }
    frame "Clear All References" {
      n101 = for {
        N: 2 -> [_]
        tunnel: [w279] -> w275 mode=indexing
        i -> [w278]
        n102 = Increment(x=w278) -> (x+1=w277:i32)
        n103 = Bundle By Name(cluster=T4 {"AlliGator Q Event"=enum."Phasor Ratio:Clear Reference n", "Data"=variant} ("element"), "Data"=w277) -> (w279:T4)
      }
      n104 = Build Array (concatenate)(w275, T4 {"AlliGator Q Event"=enum."Phasor Plot:Update Phasor Plot Reference", "Data"=variant} ("element")) -> (w273:T4[])
    }
    frame "Save References" {
    }
    frame "Load References" {
    }
    frame "Export Reference 1 to Notebook" {
      n105 = Bundle By Name(cluster=T4 {"AlliGator Q Event"=enum."Phasor Ratio:Send Reference n to Notebook", "Data"=variant} ("element"), "Data"=1) -> (w287:T4)
      n106 = Build Array(w287) -> (w285:T4[])
    }
    frame "Export Reference 2 to Notebook" {
      n107 = Bundle By Name(cluster=T4 {"AlliGator Q Event"=enum."Phasor Ratio:Send Reference n to Notebook", "Data"=variant} ("element"), "Data"=2) -> (w292:T4)
      n108 = Build Array(w292) -> (w290:T4[])
    }
    frame "Show References" {
      w304 = AlliGator_Settings_List."Phasor Plot:Show References" ("AlliGator Settings List")
      n109 = call "AlliGator Settings Storage.vi"("AlliGator Settings List"=w304, "Error In"=w297) -> ("Error Out"=w305:errorcluster, "Variant Data out"=w303:variant)  [unwired: 8 in]
      n110 = call-poly "Variant to Data.vi"("Variant"=w303) -> ("Value"=w302:bool)  [unwired: 8 in]
      n111 = Not(x=w302) -> (.not. x?=w301:bool)
      n112 = call "AlliGator Settings Storage.vi"("Get(F)/Set"=TRUE, "AlliGator Settings List"=w304, "Error In"=w305, "Variant Data in"=w301) -> ("Error Out"=w295:errorcluster)  [unwired: 6 in, 1 out]
      n113 = Bundle By Name(cluster=T4 {"AlliGator Q Event"=enum."Phasor Plot:Build Phasor Plot", "Data"=variant} ("Time-Gated Phasor Q Element"), "Data"=string[] ["Phasor Ratio References"]) -> (w299:T4)
      n114 = Build Array(w299) -> (w296:T4[])
    }
    frame "-------------------" {
    }
    frame "Zoom to Fit" {
      n115 = call "Image Display Zoom to Fit.vi"("Error In"=w309, "Keep Aspect Ratio (T)"=FALSE, "Display Image Control Refnum"=w311) -> ("Error Out"=w308:errorcluster)  [unwired: 8 in]
    }
    frame "Zoom to Fit (Keep Aspect Ratio)" {
      n116 = call "Image Display Zoom to Fit.vi"("Error In"=w313, "Display Image Control Refnum"=w314) -> ("Error Out"=w312:errorcluster)  [unwired: 9 in]
    }
  }
  "Error Out" <- w7
  "AlliGator Actions" <- w9
  "Message" <- w1
